vi "Create Command Data.vi"(4 "Command":T1, 5 "Value":u8) -> (7 "Byte":u8 format="%.0x")   [LabVIEW 2020, in "CTI-Visa-DeviceLib.lvlib" / "LCD-I2C.lvclass"]
uses:
  LCD-I2C.lvclass
  Command.ctl
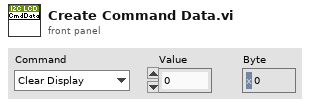
[diagram p1: front panel]
types:
  T1 = typedef "CTI-Visa-DeviceLib.lvlib/LCD-I2C.lvclass/Command.ctl" = enum16{"Clear Display", "Return Home", "Entry Mode Set", "Display Control", "Cursor Shift", "Function Set", "Set CGRAM Addr", "Set DDRAM Addr"}
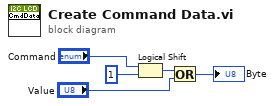
[diagram p0: block diagram]
diagram:
  n1 = Logical Shift(y="Command", x=u8 1 ("Value")) -> (x << y=w3:u8)
  n2 = Or(x=w3, y="Value") -> (x .or. y?=→"Byte":u8)
